vi "对称性补点国标算法.vi"(10 "检测点":dbl[](array[numeric]), 11 "XY图":cluster{dbl[], dbl[]}[](graph)) -> (3 "对称性":dbl[](array[numeric]))   [LabVIEW 2017]
uses:
  <vilib>/Analysis/NI_AAL_Geometry.lvlib
panel:
  out "右":dbl[](array[numeric])
  out "左":dbl[](array[numeric])
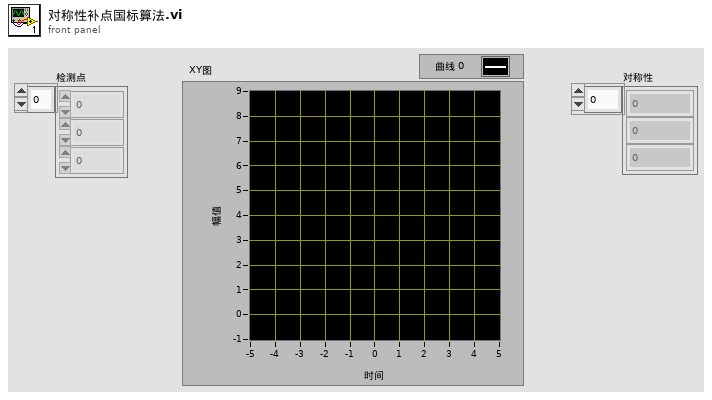
[diagram p1: front panel]
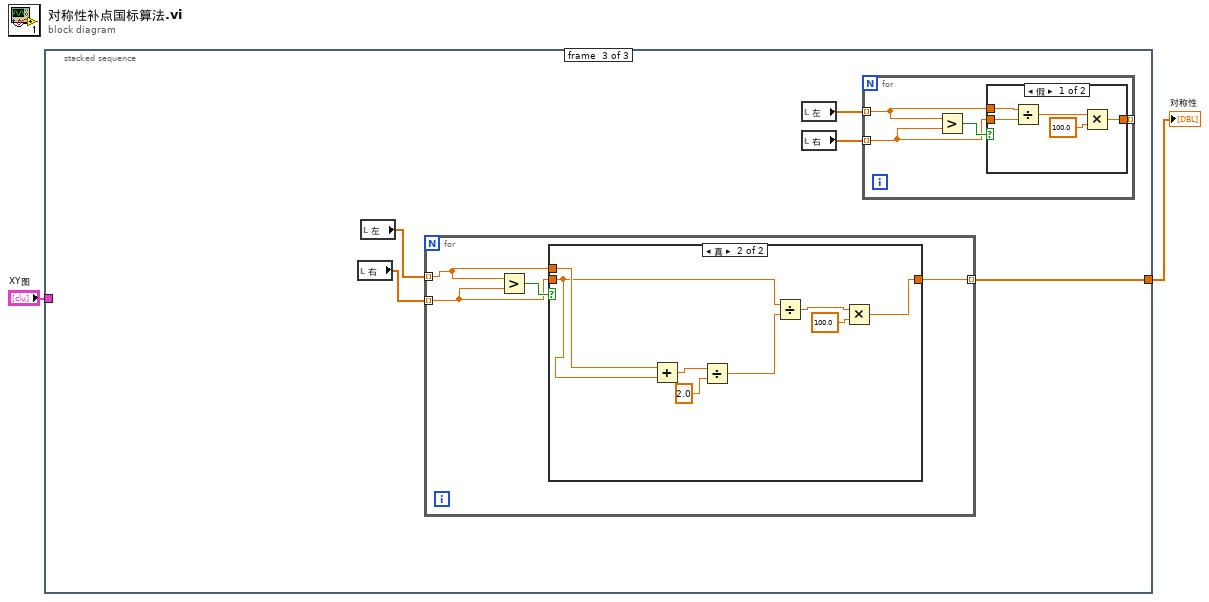
[diagram p0: block diagram]
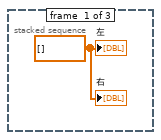
[diagram p2: hidden frame]
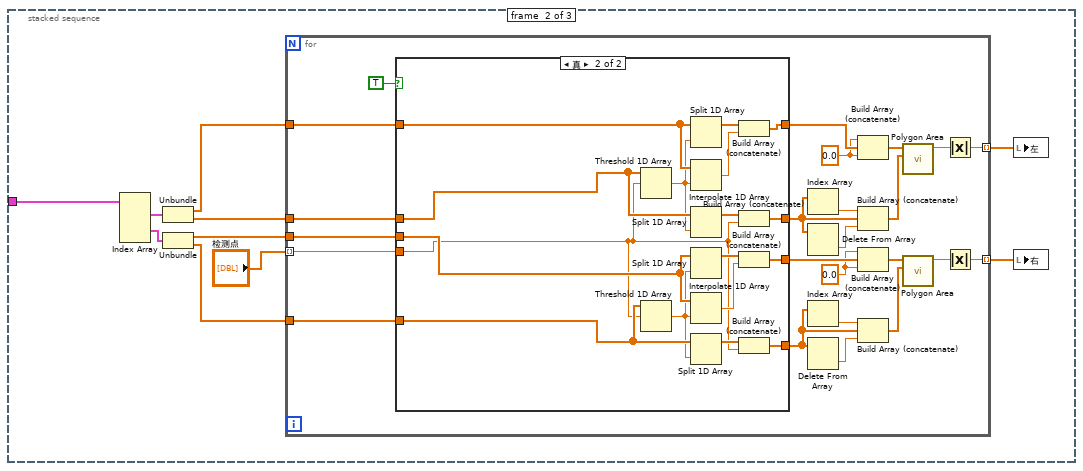
[diagram p3: hidden frame]
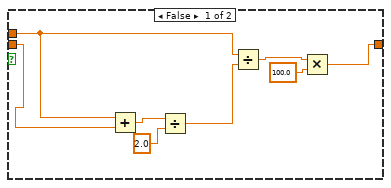
[diagram p5: hidden frame]
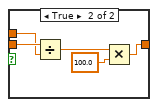
[diagram p6: hidden frame]
diagram:
  n1 = stacked-sequence {
    tunnel: "XY图" -> [_ w13 _]
    tunnel: [_ _ w59] -> w1
    frame #0 {
      w3 = dbl[] [] ("左")
      "左" <- w3
      "右" <- w3
    }
    frame #1 {
      n2 = Index Array(array=w13) -> (element #1=w6:cluster{dbl[], dbl[]}, element #3=w4:cluster{dbl[], dbl[]})  [unwired: 4 in, 2 out]
      n3 = Unbundle(w6) -> (w12:dbl[], w9:dbl[])
      n4 = Unbundle(w4) -> (w10:dbl[], w11:dbl[])
      n5 = for {
        tunnel: w12 -> [w35]
        tunnel: w11 -> [w34]
        tunnel: w10 -> [w33]
        tunnel: w9 -> [w32]
        tunnel: [w22] -> w8 mode=indexing
        tunnel: [w21] -> w7 mode=indexing
        tunnel: "检测点" -> [w14] mode=indexing
        w17 = 0.0
        w18 = 0.0
        n6 = case shown="真" TRUE {
          tunnel: w35 -> [w41 w51]
          tunnel: w34 -> [w38 w57]
          tunnel: w33 -> [w39 w46]
          tunnel: w32 -> [w40 w58]
          tunnel: [w41 w52] -> w31
          tunnel: [w40 w48] -> w29
          tunnel: [w38 w43] -> w25
          tunnel: [w39 w47] -> w24
          tunnel: w14 -> [_ w42]
          frame False {
          }
          frame True {
            n7 = Threshold 1D Array(2:w42, 3:w58) -> (0:w50:dbl)  [unwired: 1 in]
            n8 = Threshold 1D Array(2:w42, 3:w57) -> (0:w45:dbl)  [unwired: 1 in]
            n9 = Split 1D Array(array=w51, index=w50) -> (first subarray=w56:dbl[])  [unwired: 1 out]
            n10 = Interpolate 1D Array(1:w50, 2:w51) -> (0:w49:dbl)
            n11 = Split 1D Array(array=w58, index=w50) -> (first subarray=w55:dbl[])  [unwired: 1 out]
            n12 = Split 1D Array(array=w46, index=w45) -> (first subarray=w53:dbl[])  [unwired: 1 out]
            n13 = Interpolate 1D Array(1:w45, 2:w46) -> (0:w44:dbl)
            n14 = Split 1D Array(array=w57, index=w45) -> (first subarray=w54:dbl[])  [unwired: 1 out]
            n15 = Build Array (concatenate)(w56, w49) -> (w52:dbl[])
            n16 = Build Array (concatenate)(w55, w42) -> (w48:dbl[])
            n17 = Build Array (concatenate)(w53, w44) -> (w47:dbl[])
            n18 = Build Array (concatenate)(w54, w42) -> (w43:dbl[])
          }
        }
        n19 = Index Array(array=w29) -> (element=w30:dbl)  [unwired: 1 in]
        n20 = Delete From Array(array=w29) -> (deleted portion=w28:dbl)  [unwired: 2 in, 1 out]
        n21 = Index Array(array=w25) -> (element=w26:dbl)  [unwired: 1 in]
        n22 = Delete From Array(array=w25) -> (deleted portion=w27:dbl)  [unwired: 2 in, 1 out]
        n23 = Build Array (concatenate)(w18, w31, w18) -> (w20:dbl[])
        n24 = Build Array (concatenate)(w30, w29, w28) -> (w15:dbl[])
        n25 = Build Array (concatenate)(w17, w24, w17) -> (w16:dbl[])
        n26 = Build Array (concatenate)(w26, w25, w27) -> (w19:dbl[])
        n27 = call <vilib>:"Polygon Area.vi"("Y"=w15, "X"=w20) -> ("signed area"=w36:dbl)  [unwired: 8 in, 1 out]
        n28 = call <vilib>:"Polygon Area.vi"("Y"=w19, "X"=w16) -> ("signed area"=w37:dbl)  [unwired: 8 in, 1 out]
        n29 = Absolute Value(x=w36) -> (abs(x)=w22:dbl)
        n30 = Absolute Value(x=w37) -> (abs(x)=w21:dbl)
      }
      n31 = local write "左"(w8) -> ()
      n32 = local write "右"(w7) -> ()
    }
    frame #2 {
      n33 = local read "右"() -> (w60:dbl[])
      n34 = local read "左"() -> (w61:dbl[])
      n35 = for {
        tunnel: w60 -> [w66] mode=indexing
        tunnel: [w65] -> w59 mode=indexing
        tunnel: w61 -> [w64] mode=indexing
        n36 = Greater?(x=w64, y=w66) -> (0:w67:bool)
        n37 = case shown="真" w67 {
          tunnel: w66 -> [w69 w76]
          tunnel: w64 -> [w68 w80]
          tunnel: [w71 w81] -> w65
          frame False {
            n38 = Add(x=w68, y=w69) -> (x+y=w74:dbl)
            n39 = Divide(x=w74, y=2.0) -> (x/y=w72:dbl)
            n40 = Divide(x=w68, y=w72) -> (x/y=w70:dbl)
            n41 = Multiply(x=w70, y=100.0) -> (x*y=w71:dbl)
          }
          frame True {
            n42 = Add(x=w80, y=w76) -> (x+y=w79:dbl)
            n43 = Divide(x=w79, y=2.0) -> (x/y=w77:dbl)
            n44 = Divide(x=w76, y=w77) -> (x/y=w82:dbl)
            n45 = Multiply(x=w82, y=100.0) -> (x*y=w81:dbl)
          }
        }
      }
      n46 = local read "左"() -> (w62:dbl[])
      n47 = local read "右"() -> (w63:dbl[])
      n48 = for {
        tunnel: w63 -> [w86] mode=indexing
        tunnel: w62 -> [w85] mode=indexing
        tunnel: [w84] -> _ mode=indexing
        n49 = Greater?(x=w85, y=w86) -> (0:w87:bool)
        n50 = case shown="假" w87 {
          tunnel: w86 -> [w91 w97]
          tunnel: w85 -> [w92 w96]
          tunnel: [w88 w94] -> w84
          frame False {
            n51 = Divide(x=w92, y=w91) -> (x/y=w90:dbl)
            n52 = Multiply(x=w90, y=100.0) -> (x*y=w88:dbl)
          }
          frame True {
            n53 = Divide(x=w97, y=w96) -> (x/y=w95:dbl)
            n54 = Multiply(x=w95, y=100.0) -> (x*y=w94:dbl)
          }
        }
      }
    }
  }
  "对称性" <- w1
